vi "swabian_initialize_log_histogram.vi"(8 "error in (no error)":errorcluster, 9 "acq_time":i64 min=0, 10 "histo-settings":T1={"start_time(10^s)"=0.0, "stop_time(10^s)"=0.0, "start_channel"=enum."No Selection", "stop-channel"=enum."No Selection", "n_bins"=0, "Channels to\nHistogram"=[FALSE, FALSE, FALSE, FALSE, FALSE, FALSE, FALSE, FALSE]}, 11 "swabian_local_data":T3={"events"={"update_status"=refnum, "update_chart"=refnum, "update_xy"=refnum, "send_channel_data"=refnum}, "stop_q"=refnum, "tagger_reference"=refnum, "connect_button"=refnum, "counter_reference"=refnum, "tagger_stream_reference"=refnum, "log_reference"=refnum, "current_log_offset"=0, "tt20_buffer_q"=refnum, "stream_to_file_button"=refnum, "num_records"=0, "connected?"=FALSE, "plots"=refnum, "histogram_bin_edges"=[], "histogrammer"=refnum, "plot_lifetimes"=refnum, "xy_graph"=refnum, "Reference\nChannel"=enum."ch0"}) -> (0 "error out":errorcluster, 3 "swabian_local_data 2":T3={"events"={"update_status"=refnum, "update_chart"=refnum, "update_xy"=refnum, "send_channel_data"=refnum}, "stop_q"=refnum, "tagger_reference"=refnum, "connect_button"=refnum, "counter_reference"=refnum, "tagger_stream_reference"=refnum, "log_reference"=refnum, "current_log_offset"=0, "tt20_buffer_q"=refnum, "stream_to_file_button"=refnum, "num_records"=0, "connected?"=FALSE, "plots"=refnum, "histogram_bin_edges"=[], "histogrammer"=refnum, "plot_lifetimes"=refnum, "xy_graph"=refnum, "Reference\nChannel"=enum."ch0"})   [LabVIEW 2015]
uses:
  swabian_local_data_tdef.ctl
  swabian_events_tdef.ctl
  update_chart_tdef.ctl
  channel_data_tdef.ctl
  C:/Users/bspoka/Dropbox (MIT)/Swabian/lib/TTCSharp32.dll
  lib/TTCSharp32.dll
  swabian_buffer_tdef.ctl
  reference_checkbox_tdef.ctl
  swabian_hisotgram_settings.ctl
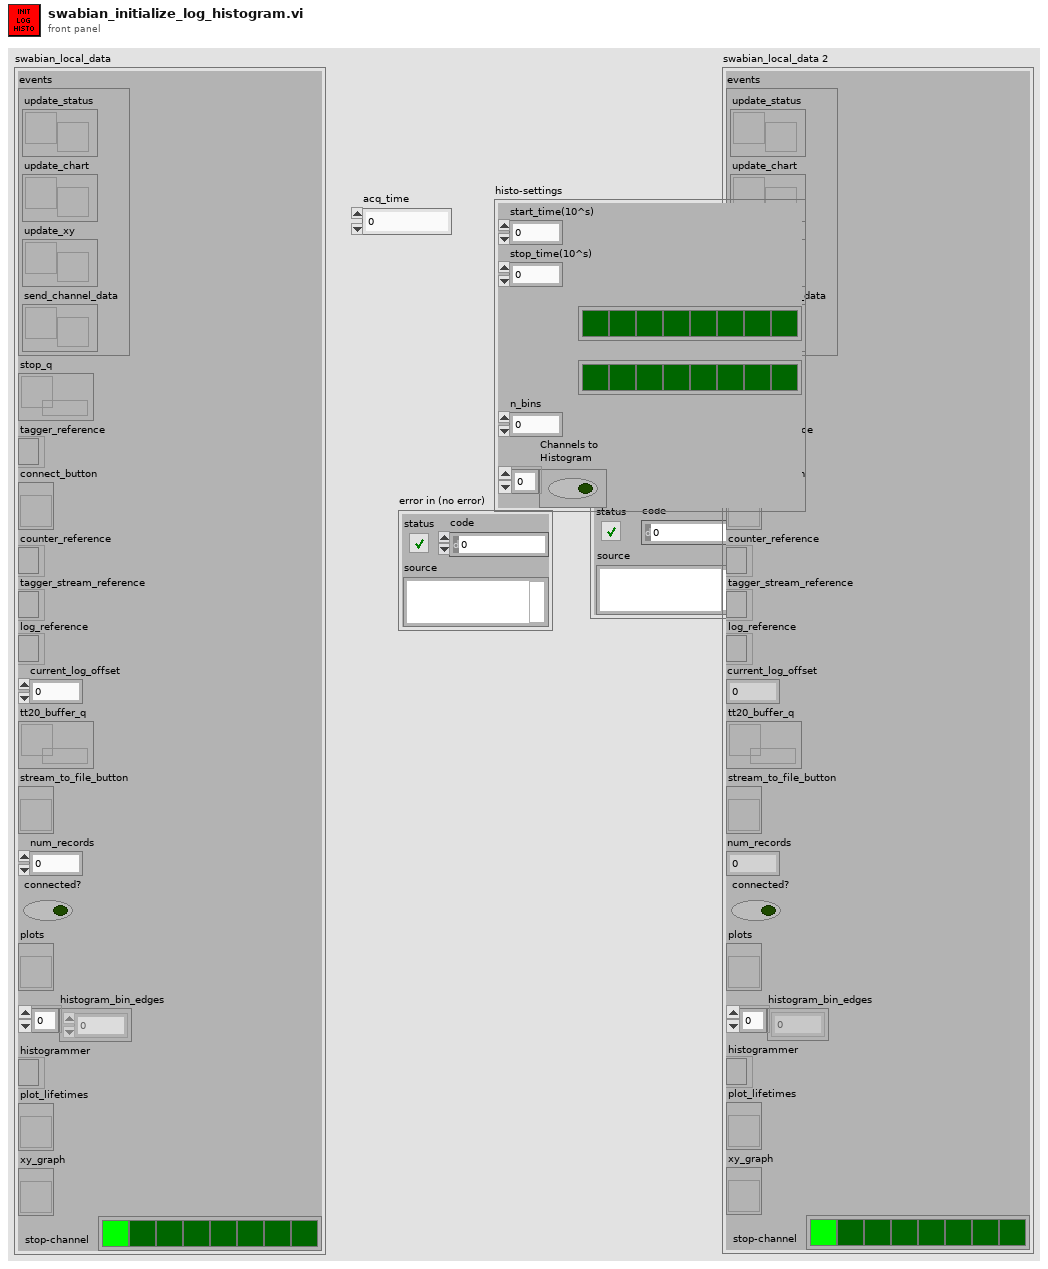
[diagram p1: front panel]
types:
  T1 = typedef "swabian_hisotgram_settings.ctl" = cluster{"start_time(10^s)":dbl, "stop_time(10^s)":dbl, "start_channel":T2, "stop-channel":T2, "n_bins":i32, "Channels to\nHistogram":bool[]}
  T2 = typedef "reference_checkbox_tdef.ctl" = enum32{"No Selection", "ch0", "ch1", "ch2", "ch3", "ch4", "ch5", "ch6", "ch7"}
  T3 = typedef "swabian_local_data_tdef.ctl" = cluster{"events":T4, "stop_q":refnum<queue>, "tagger_reference":refnum<k24>, "connect_button":refnum<vi>, "counter_reference":refnum<k24>, "tagger_stream_reference":refnum<k24>, "log_reference":refnum<file>, "current_log_offset":i64, "tt20_buffer_q":refnum<queue>, "stream_to_file_button":refnum<vi>, "num_records":u64, "connected?":bool, "plots":refnum<vi>, "histogram_bin_edges":i64[], "histogrammer":refnum<k24>, "plot_lifetimes":refnum<vi>, "xy_graph":refnum<vi>, "Reference\nChannel":T2}
  T4 = typedef "swabian_events_tdef.ctl" = cluster{"update_status":refnum<user-event>, "update_chart":refnum<user-event>, "update_xy":refnum<user-event>, "send_channel_data":refnum<user-event>}
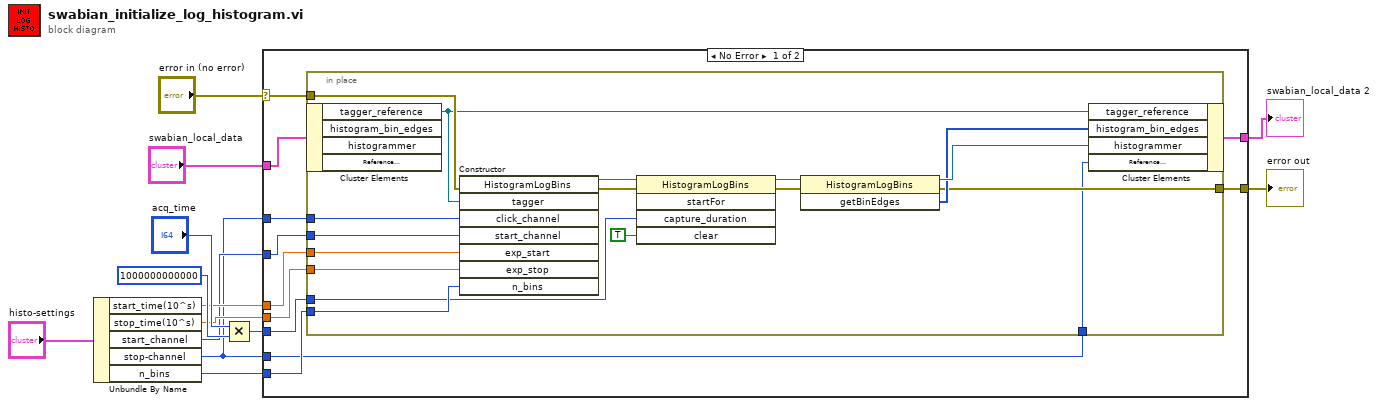
[diagram p0: block diagram]
diagram:
  n1 = Unbundle By Name("histo-settings") -> ("start_time(10^s)"=w5:dbl, "stop_time(10^s)"=w4:dbl, "start_channel"=w2:T2, "stop-channel"=w1:T2, "n_bins"=w3:i32)
  n2 = Multiply(x="acq_time", y=i64 1000000000000) -> (x*y=w7:i64)
  n3 = case shown="No Error" "error in (no error)" {
    selector: "error in (no error)" -> [w18 w42]
    tunnel: "swabian_local_data" -> [w24 w43]
    tunnel: w2 -> [w23 _]
    tunnel: w7 -> [w17 _]
    tunnel: [w16 w42] -> w13
    tunnel: [w15 w43] -> w12
    tunnel: w1 -> [w22 _]
    tunnel: w5 -> [w21 _]
    tunnel: w4 -> [w20 _]
    tunnel: w3 -> [w19 _]
    tunnel: w1 -> [w14 _]
    frame No Error {
      n4 = in-place {
        in-place-border: w23 -> [w41]
        in-place-border: w22 -> [w40]
        in-place-border: w21 -> [w39]
        in-place-border: w20 -> [w38]
        in-place-border: w19 -> [w37]
        in-place-border: w18 -> [w36]
        in-place-border: w17 -> [w31]
        in-place-border: [w26] -> w16
        in-place-border: w14 -> [w25]
        n5 = in-place-cluster #1(w24) -> ("tagger_reference"=w27:refnum<k24>)  [unwired: 3 out]
        n6 = constructor class="HistogramLogBins"(error in=w36, "tagger"=w27, "click_channel"=w40, "start_channel"=w41, "exp_start"=w39, "exp_stop"=w38, "n_bins"=w37) -> (reference out=w35:refnum<k24>, error out=w29:errorcluster)  [unwired: 2 in, 7 out]
        n7 = invoke class="HistogramLogBins" method="startFor"(reference=w35, error in=w29, "capture_duration"=w31, "clear"=TRUE) -> (reference out=w34:refnum<k24>, error out=w28:errorcluster)  [unwired: 1 in, 3 out]
        n8 = invoke class="HistogramLogBins" method="getBinEdges"(reference=w34, error in=w28) -> (reference out=w33:refnum<k24>, error out=w26:errorcluster, "getBinEdges"=w32:i64[])  [unwired: 1 in]
        n9 = in-place-cluster #1("tagger_reference"=w27, "histogram_bin_edges"=w32, "histogrammer"=w33, "Reference\nChannel"=w25) -> (w15:T3)
      }
    }
    frame Error {
    }
  }
  "swabian_local_data 2" <- w12
  "error out" <- w13
